vi "Generator_and_Motor.vi"(8 "Initialize":bool, 9 "Speed":dbl, 10 "Speed Voltage Factor":dbl, 11 "Motor Load":dbl) -> (2 "Motor Speed":dbl, 3 "Motor Torque":dbl)   [LabVIEW 2020]
uses:
  <vilib>/Simulation/Scripting/Companion Diagram/SimConfigNode/SimParams.ctl
  <vilib>/Simulation/Scripting/Companion Diagram/SimConfigNode/_simSolvers.ctl
  <vilib>/Simulation/Implementation/Shared/SIMSCR Execution Mode.ctl
  <vilib>/Simulation/Param Hierarchy/Typedefs/SIMPH Param Control Actions.ctl
  <vilib>/Simulation/Implementation/Shared/NILVSim_ParamChanged.vi
  <vilib>/Simulation/Implementation/Shared/NILVSIM_BeginStep.vi
  <vilib>/Simulation/Implementation/Shared/NILVSim_Manager.vi
  <vilib>/Utility/error.llb/Clear Errors.vi
  <vilib>/Simulation/Implementation/Shared/NILVSim_FinalizeModel.vi
  <vilib>/Simulation/Implementation/Shared/SIM Unbundle Sim Info.vi
  <vilib>/Simulation/Implementation/Shared/NILVSim_Initialize.vi
  <vilib>/Simulation/Utility/Implementation/NILVSim Get Time and IsAcceptedStep.vi
  <vilib>/Simulation/Implementation/Shared/SIMSH Read Queue.vi
  <vilib>/Simulation/Implementation/Shared/NILVSim_GetModelError.vi
  <vilib>/Simulation/Implementation/Shared/SIM Bundle Sim Info.vi
  <vilib>/Simulation/Implementation/XNodeFramework/SimXNode/SimX.xnode
  C:/Program Files/National Instruments/LabVIEW 2020/examples/Control and Simulation/Case Studies/Electrical Machines/DC Motor/SimEx DC Motor Model.vi
  <vilib>/Simulation/Scripting/Companion Diagram/SimConfigNode/SimDog.xnode
  <vilib>/Simulation/Implementation/Shared/NI_SIM_Implementation.lvlib
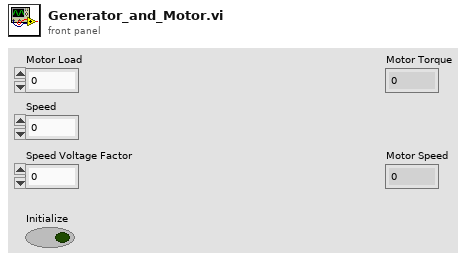
[diagram p1: front panel]
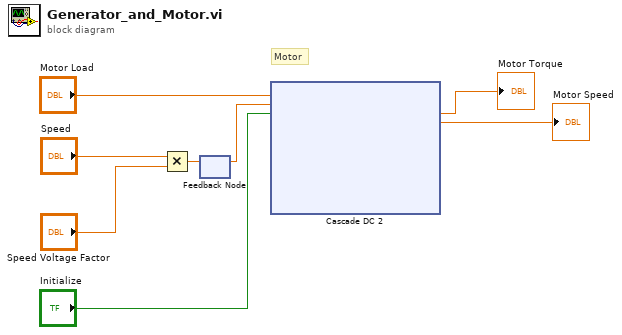
[diagram p0: block diagram]
diagram:
  # "Motor"
  n1 = Multiply(x="Speed", y="Speed Voltage Factor") -> (x*y=w6:dbl)
  n2 = feedback #1() -> (w7:dbl)  [unwired: 1 in]
  n3 = feedback-in #1(w6) -> ()
  n4 = xnode ("Cascade DC 2")("TL"="Motor Load", "voltage"=w7, "Initialize"="Initialize") -> ("Te"=→"Motor Torque":dbl, "Speed"=→"Motor Speed":dbl)  [unwired: 1 in, 6 out]
